vi "czesc5.vi"   [LabVIEW 2022 SP3]
types:
  T1 = enum16{"open", "replace", "create", "open or create", "replace or create", "replace or create with confirmation"}
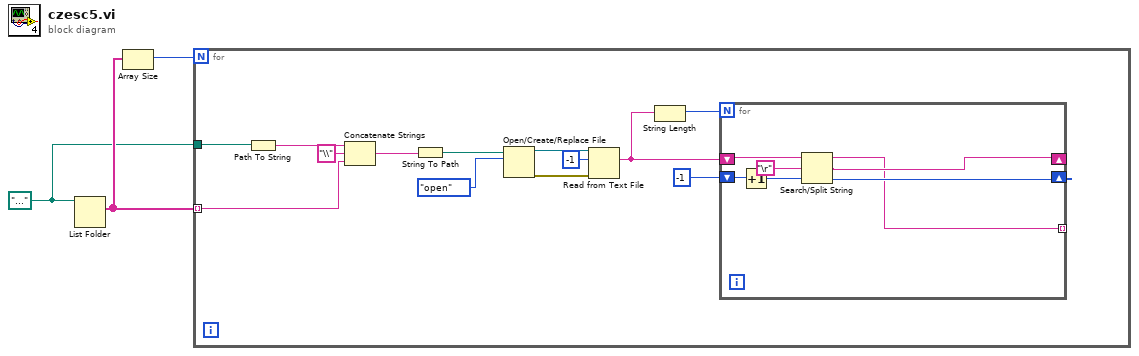
[diagram p0: block diagram]
diagram:
  w1 = path "..." ("file path (use dialog)")
  n1 = List Folder(path=w1) -> (filenames=w2:string[])  [unwired: 3 in, 3 out]
  n2 = Array Size(array=w2) -> (size(s)=w3:i32)
  n3 = for {
    N: w3 -> [_]
    tunnel: w2 -> [w13] mode=indexing
    tunnel: w1 -> [w16]
    n4 = Path To String(path=w16) -> (string=w15:string)
    n5 = Concatenate Strings(w15, "\\" ("string"), w13) -> (w12:string)
    n6 = String To Path(string=w12) -> (path=w11:path)
    n7 = Open/Create/Replace File(file path (use dialog)=w11, operation (0:open)=T1."open") -> (refnum out=w9:refnum<file>, error out=w7:errorcluster)  [unwired: 4 in, 1 out]
    n8 = Read from Text File(file (use dialog)=w9, count=-1, error in=w7) -> (text=w5:string)  [unwired: 1 in, 3 out]
    n9 = String Length(string=w5) -> (length=w6:i32)
    n10 = for {
      N: w6 -> [_]
      shift-right: [w18] -> _
      shift-left: w5 -> [w22]
      shift-right: [w19] -> _
      shift-left: -1 -> [w20]
      tunnel: [w17] -> _ mode=indexing
      n11 = Increment(x=w20) -> (x+1=w19:i32)
      n12 = Search/Split String(string=w22, search string/char (-)="\r", offset (0)=w19) -> (substring before match=w17:string, match + rest of string=w18:string)  [unwired: 1 out]
    }
  }
